vi "Load Control Info.vi"(7 "BG Color (Dark Gray)":u32(colorbox)=2631720, 8 "error in (no error)":errorcluster, 10 "Control Path":path) -> (0 "error out":errorcluster, 2 "Info":T1)   [LabVIEW 2020, in "VolatusGUIEditor.lvlib"]
uses:
  VolatusGUIEditor.lvlib
  Control Info.ctl
  <vilib>/picture/picture.llb/imagedata.ctl
  lv-volatus/VolatusGUI/VolatusGUI.lvlib
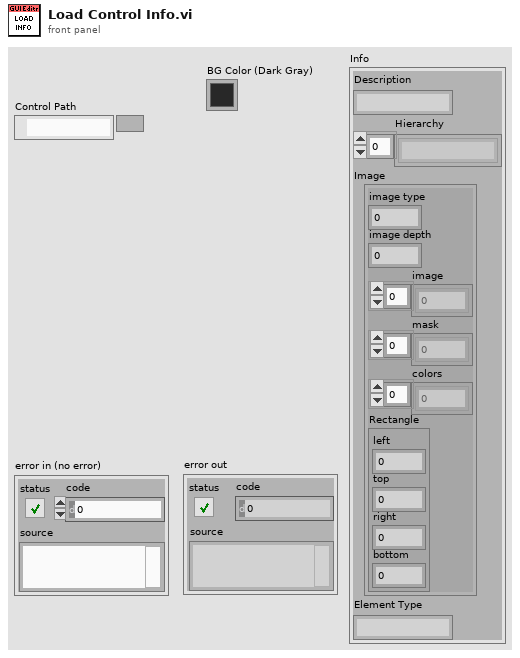
[diagram p1: front panel]
types:
  T1 = typedef "VolatusGUIEditor.lvlib/Control Info.ctl" = cluster{"Description":string, "Hierarchy":string[], "Image":T2, "Element Type":string}
  T2 = typedef "imagedata.ctl" = cluster{"image type":i32, "image depth":i32, "image":u8[], "mask":u8[], "colors":u32[], "Rectangle":cluster{"left":i16, "top":i16, "right":i16, "bottom":i16}}
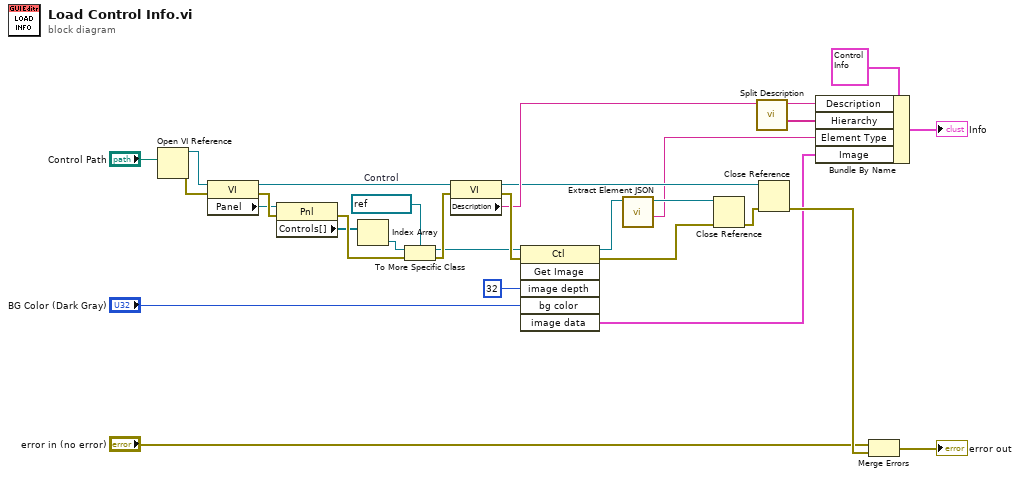
[diagram p0: block diagram]
diagram:
  w22 = refnum<vi> refnum  # Control
  n1 = Open VI Reference(vi path="Control Path") -> (vi reference=w26:refnum<vi>, error out=w27:errorcluster)  [unwired: 5 in]
  n2 = property class="VI"(reference=w26, error in=w27) -> (reference out=w10:refnum<vi>, error out=w28:errorcluster, "Panel"=w25:refnum<vi>)
  n3 = property class="Pnl"(reference=w25, error in=w28) -> (error out=w29:errorcluster, "Controls[]"=w24:refnum<vi>[])  [unwired: 1 out]
  n4 = Index Array(array=w24) -> (element=w23:refnum<vi>)  [unwired: 1 in]
  n5 = To More Specific Class(target class=w22, reference=w23, error in=w29) -> (specific class reference=w7:refnum<vi>, error out=w9:errorcluster)
  n6 = property class="VI"(reference=w10, error in=w9) -> (reference out=w5:refnum<vi>, error out=w8:errorcluster, "Description"=w6:string)
  n7 = invoke class="Ctl" method="Get Image"(reference=w7, error in=w8, "image depth"=32 ("Image Depth"), "bg color"="BG Color (Dark Gray)") -> (reference out=w4:refnum<vi>, error out=w2:errorcluster, "image data"=w17:T2)  [unwired: 2 in, 3 out]
  n8 = call "Extract Element JSON.vi"("Ctl Refnum in"=w4) -> ("Type"=w1:string, "Ctl Refnum"=w3:refnum<vi>)  [unwired: 7 in, 2 out]
  n9 = Close Reference(reference=w3, error in (no error)=w2) -> (error out=w11:errorcluster)
  n10 = call "Split Description.vi"("Full Description"=w6) -> ("Description"=w16:string, "Hierarchy"=w15:string[])  [unwired: 9 in]
  n11 = Close Reference(reference=w5, error in (no error)=w11) -> (error out=w30:errorcluster)
  n12 = Bundle By Name(cluster=T1 {"Description"="", "Hierarchy"=[], "Image"={"image type"=0, "image depth"=0, "image"=[], "mask"=[], "colors"=[], "Rectangle"={"left"=0, "top"=0, "right"=0, "bottom"=0}}, "Element Type"=""} ("Control Info"), "Description"=w16, "Hierarchy"=w15, "Element Type"=w1, "Image"=w17) -> (→"Info":T1)
  n13 = Merge Errors("error in (no error)", w30) -> (→"error out":errorcluster)
